vi "1WIRE_READ_SCRATCHPAD.vi"(6 "1-Wire DIO Pin":refnum<k21>="ConnectorA/DIO15", 7 "error in (no error)":errorcluster) -> (0 "error out":errorcluster, 2 "Scratchpad Data":u8[](array[numeric]) format="%.0x")   [LabVIEW 2014]
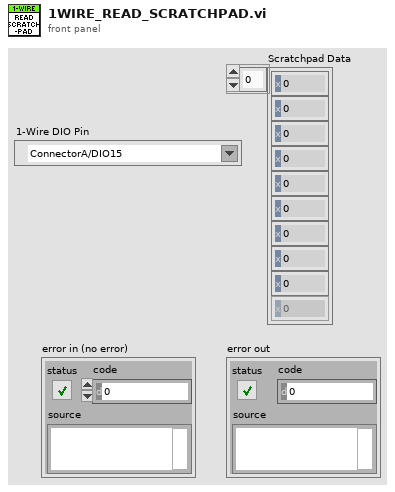
[diagram p1: front panel]
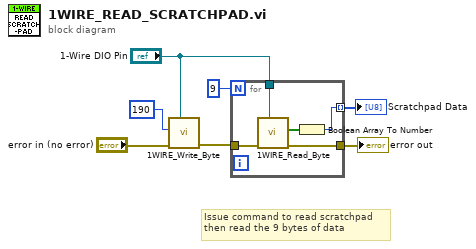
[diagram p0: block diagram]
diagram:
  # "Issue command to read scratchpad\nthen read the 9 bytes of data"
  n1 = call "1WIRE_Write_Byte.vi"("1-Wire DIO Pin"="1-Wire DIO Pin", "error in"="error in (no error)", "Tx data"=u8 190 ("Tx data 2")) -> ("error out"=w4:errorcluster)  [unwired: 7 in, 1 out]
  n2 = for {
    N: 9 -> [_]
    tunnel: w4 -> [w12]
    tunnel: [w11] -> w6
    tunnel: [w9] -> w2 mode=indexing
    tunnel: "1-Wire DIO Pin" -> [w8]
    n3 = call "1WIRE_Read_Byte.vi"("1-Wire DIO Pin"=w8, "error in"=w12) -> ("error out"=w11:errorcluster, "Array"=w10:bool[])  [unwired: 8 in]
    n4 = Boolean Array To Number(Boolean array=w10) -> (number=w9:u8)
  }
  "Scratchpad Data" <- w2
  "error out" <- w6
